vi "Lakeshore 336 Big Temp Read.vi"(8 "error in (no error)":errorcluster, 10 "Read Which Value?":enum32{"Sorb", "1K Pot", "He3 Pot", "Probe"}(ring), 11 "VISA Refnum in":refnum<visa-resource-name>) -> (0 "error out":errorcluster, 2 "Measurement":dbl[](array[numeric]), 3 "VISA Refnum out":refnum<visa-resource-name>)   [LabVIEW 2020]
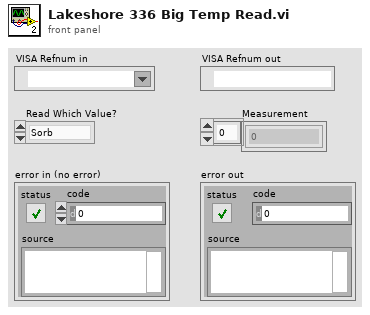
[diagram p1: front panel]
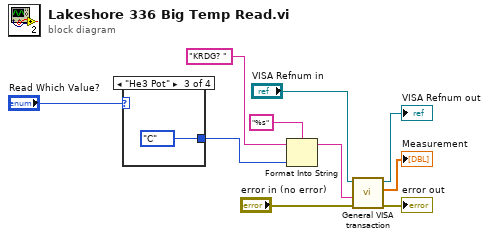
[diagram p0: block diagram]
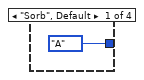
[diagram p2: hidden frame]
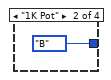
[diagram p3: hidden frame]
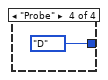
[diagram p4: hidden frame]
diagram:
  n1 = case shown="\"He3 Pot\"" "Read Which Value?" {
    tunnel: [enum16{"A", "B", "C", "D"}."A" ("LakeShore 340 Channel") enum16{"A", "B", "C", "D"}."B" ("LakeShore 340 Channel") enum16{"A", "B", "C", "D"}."C" ("LakeShore 340 Channel") enum16{"A", "B", "C", "D"}."D" ("LakeShore 340 Channel")] -> w10
    frame "Sorb", Default {
    }
    frame "1K Pot" {
    }
    frame "He3 Pot" {
    }
    frame "Probe" {
    }
  }
  n2 = Format Into String(format string="%s", initial string="KRDG? " ("Format String"), w10) -> (resulting string=w4:string)  [unwired: 1 in, 1 out]
  n3 = call "General VISA transaction.vi"("error in (no error)"="error in (no error)", "Command String"=w4, "VISA Session"="VISA Refnum in") -> ("error out"=→"error out":errorcluster, "Measurement"=→"Measurement":dbl[], "dup VISA Session"=→"VISA Refnum out":refnum<visa-resource-name>)  [unwired: 3 in, 3 out]
